vi "Statistics.vi"(7 "error in (no error)":errorcluster, 10 "Graph Data In":T1) -> (0 "error out":errorcluster, 2 "New Graph Data Out":T1)   [LabVIEW 2013, in "Diode Characterization.lvlib" / "Diode IV.lvclass"]
doc: "Computes basic statistics (mean, RMS, min, max, peak to peak and frequency) for each waveform in the input data and outputs annotations."
uses:
  Diode IV.lvclass
  graphdata.ctl
  <vilib>/Utility/miscctls.llb/LVAnnotationListTypeDef.ctl
  <vilib>/Utility/miscctls.llb/LVCursorListTypeDef.ctl
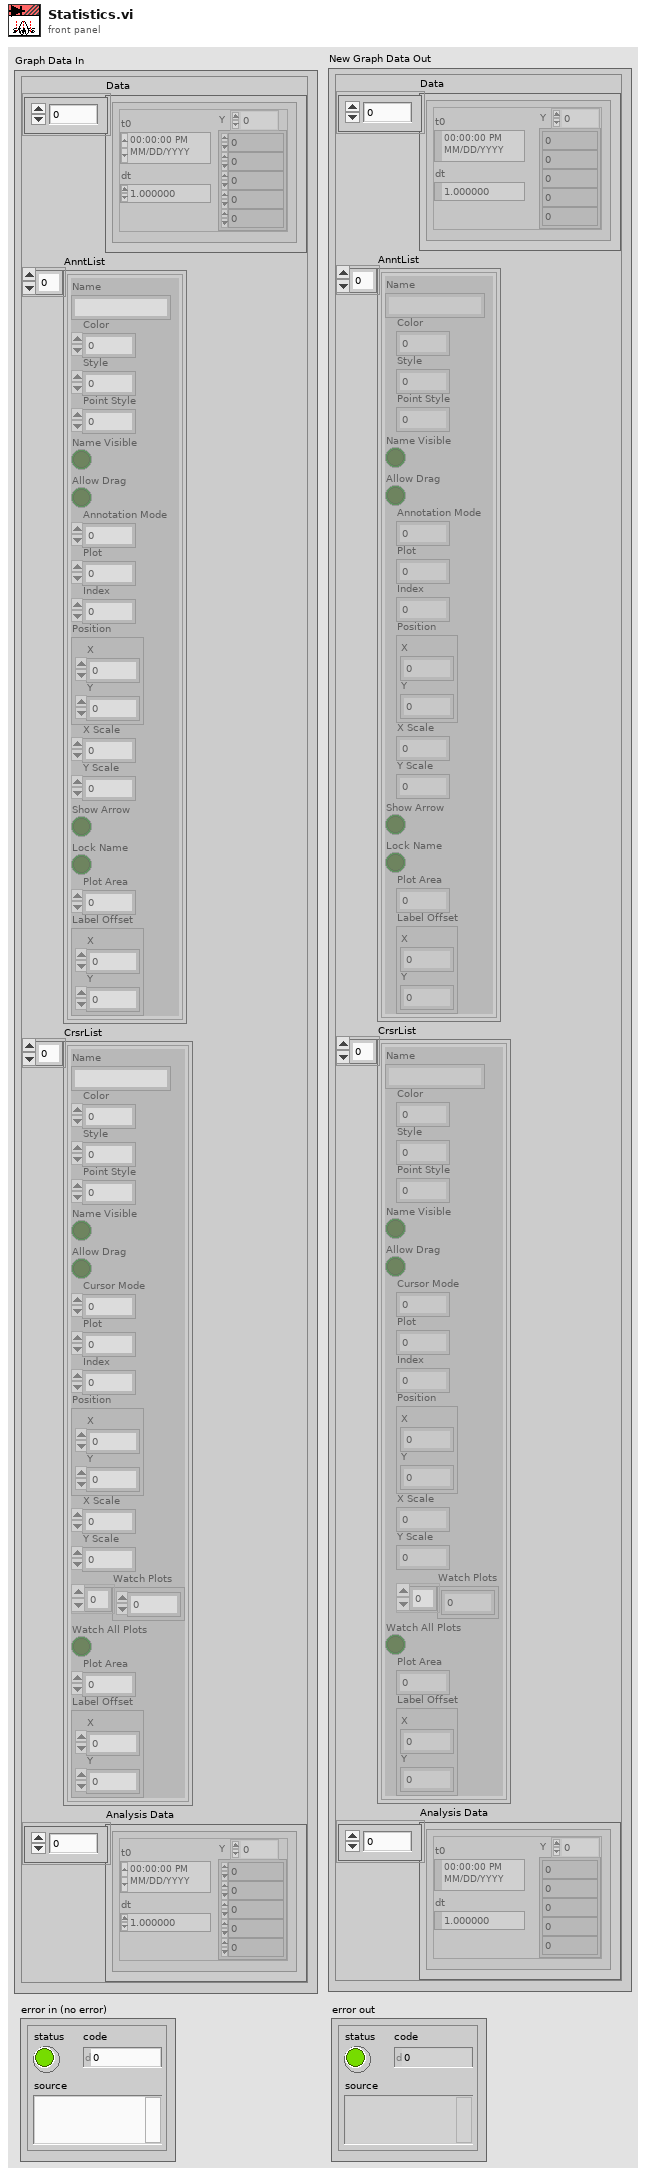
[diagram p1: front panel]
types:
  T1 = typedef "Diode Characterization.lvlib/Diode IV.lvclass/graphdata.ctl" = cluster{"Data":waveform(dbl)[], "AnntList":T2, "CrsrList":T3, "Analysis Data":waveform(dbl)[]}
  T2 = typedef "LVAnnotationListTypeDef.ctl" = cluster{"Name":string, "Color":u32, "Style":u8, "Point Style":u8, "Name Visible":bool, "Allow Drag":bool, "Annotation Mode":u32, "Plot":i32, "Index":i32, "Position":cluster{"X":dbl, "Y":dbl}, "X Scale":u32, "Y Scale":u32, "Show Arrow":bool, "Lock Name":bool, "Plot Area":i32, "Label Offset":cluster{"X":dbl, "Y":dbl}}[]
  T3 = typedef "LVCursorListTypeDef.ctl" = cluster{"Name":string, "Color":u32, "Style":u8, "Point Style":u8, "Name Visible":bool, "Allow Drag":bool, "Cursor Mode":u32, "Plot":i32, "Index":i32, "Position":cluster{"X":dbl, "Y":dbl}, "X Scale":u32, "Y Scale":u32, "Watch Plots":i32[], "Watch All Plots":bool, "Plot Area":i32, "Label Offset":cluster{"X":dbl, "Y":dbl}}[]
  T4 = cluster{"Name":string, "Color":u32, "Style":u8, "Point Style":u8, "Name Visible":bool, "Allow Drag":bool, "Annotation Mode":u32, "Plot":i32, "Index":i32, "Position":cluster{"X":dbl, "Y":dbl}, "X Scale":u32, "Y Scale":u32, "Show Arrow":bool, "Lock Name":bool, "Plot Area":i32, "Label Offset":cluster{"X":dbl, "Y":dbl}}
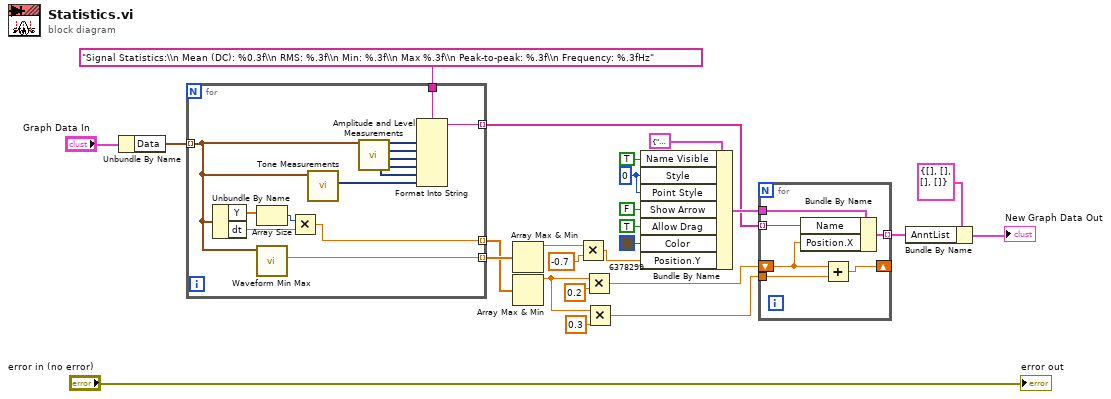
[diagram p0: block diagram]
diagram:
  w22 = u8 0 ("Style")
  n1 = Unbundle By Name("Graph Data In") -> ("Data"=w18:waveform(dbl)[])
  n2 = for {
    tunnel: w18 -> [w30] mode=indexing
    tunnel: [w39] -> w2 mode=indexing
    tunnel: "Signal Statistics:\\n Mean (DC): %0.3f\\n RMS: %.3f\\n Min: %.3f\\n Max %.3f\\n Peak-to-peak: %.3f\\n Frequency: %.3fHz" ("format string") -> [w38]
    tunnel: [w37] -> w8 mode=indexing
    tunnel: [w26] -> w1 mode=indexing
    n3 = Unbundle By Name(w30) -> ("Y"=w29:dbl[], "dt"=w27:dbl)
    n4 = Array Size(array=w29) -> (size(s)=w28:i32)
    n5 = call <vilib>:"Waveform Min Max.vi"("waveform in"=w30) -> ("Y max"=w39:dbl)  [unwired: 5 in, 5 out]
    n6 = Multiply(x=w28, y=w27) -> (x*y=w26:dbl)
    n7 = call "Tone Measurements"("Signals"=w30) -> ("Frequency"=w31:dynamicdata)  [unwired: 9 in, 1 out]
    n8 = call "Amplitude and Level Measurements"("Signals"=w30) -> ("Mean (DC)"=w36:dynamicdata, "RMS"=w35:dynamicdata, "Negative Peak"=w34:dynamicdata, "Positive Peak"=w33:dynamicdata, "Peak to Peak"=w32:dynamicdata)  [unwired: 9 in, 1 out]
    n9 = Format Into String(format string=w38, w36, w35, w34, w33, w32, w31) -> (resulting string=w37:string)  [unwired: 2 in, 1 out]
  }
  n10 = Array Max & Min(array=w2) -> (max value=w16:dbl)  [unwired: 3 out]
  n11 = Array Max & Min(array=w1) -> (max value=w10:dbl)  [unwired: 3 out]
  n12 = Multiply(x=w16, y=-0.7) -> (x*y=w14:dbl)
  n13 = Multiply(x=w10, y=0.2) -> (x*y=w12:dbl)
  n14 = Multiply(x=w10, y=0.3) -> (x*y=w11:dbl)
  n15 = Bundle By Name(cluster=T4 {"Name"="", "Color"=0, "Style"=0, "Point Style"=0, "Name Visible"=FALSE, "Allow Drag"=FALSE, "Annotation Mode"=0, "Plot"=0, "Index"=0, "Position"={"X"=0.0, "Y"=0.0}, "X Scale"=0, "Y Scale"=0, "Show Arrow"=FALSE, "Lock Name"=FALSE, "Plot Area"=0, "Label Offset"={"X"=0.0, "Y"=0.0}} ("element"), "Name Visible"=TRUE, "Style"=w22, "Point Style"=w22, "Show Arrow"=FALSE, "Allow Drag"=TRUE, "Color"=u32 6378299, "Position.Y"=w14) -> (w17:T4)
  n16 = for {
    tunnel: w17 -> [w45]
    shift-right: [w42] -> _
    shift-left: w12 -> [w44]
    tunnel: w11 -> [w43]
    tunnel: [w41] -> w7 mode=indexing
    tunnel: w8 -> [w40] mode=indexing
    n17 = Bundle By Name(cluster=w45, "Name"=w40, "Position.X"=w44) -> (w41:T4)
    n18 = Add(x=w44, y=w43) -> (x+y=w42:dbl)
  }
  n19 = Bundle By Name(cluster=T1 {"Data"=[], "AnntList"=[], "CrsrList"=[], "Analysis Data"=[]} ("Graph Data In"), "AnntList"=w7) -> (→"New Graph Data Out":T1)
  "error out" <- "error in (no error)"
